vi "Read ADC.vi"(0 "Session Handle in":T1, 11 "error in (no error)":errorcluster) -> (4 "Session Handle out":T1, 6 "ADC":dbl, 8 "Error Code":string, 10 "code":i32, 15 "error out":errorcluster)   [LabVIEW 2015, in "PAS.lvclass"]
uses:
  PAS.lvclass
  Typedefs/Session Handle.ctl
panel:
  out "Success?":bool
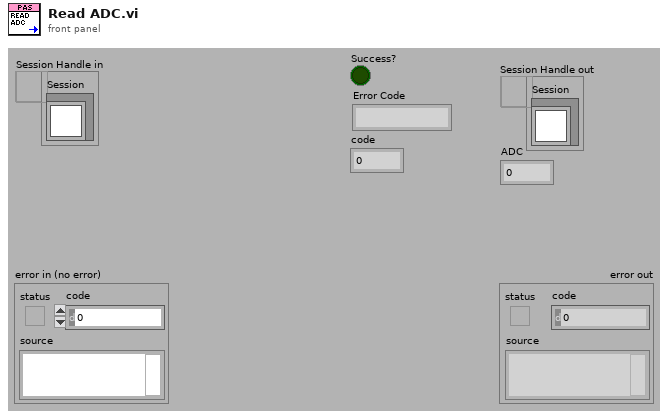
[diagram p1: front panel]
types:
  T1 = typedef "PAS.lvclass/Session Handle.ctl" = refnum<data-value>
  T2 = typedef "XNET Frame CAN.ctl" = cluster{"timestamp":timestamp, "payload":u8[], "identifier":u32, "type":T3, "extended?":bool, "echo?":bool}
  T3 = typedef "XNET Frame Type CAN.ctl" = u8
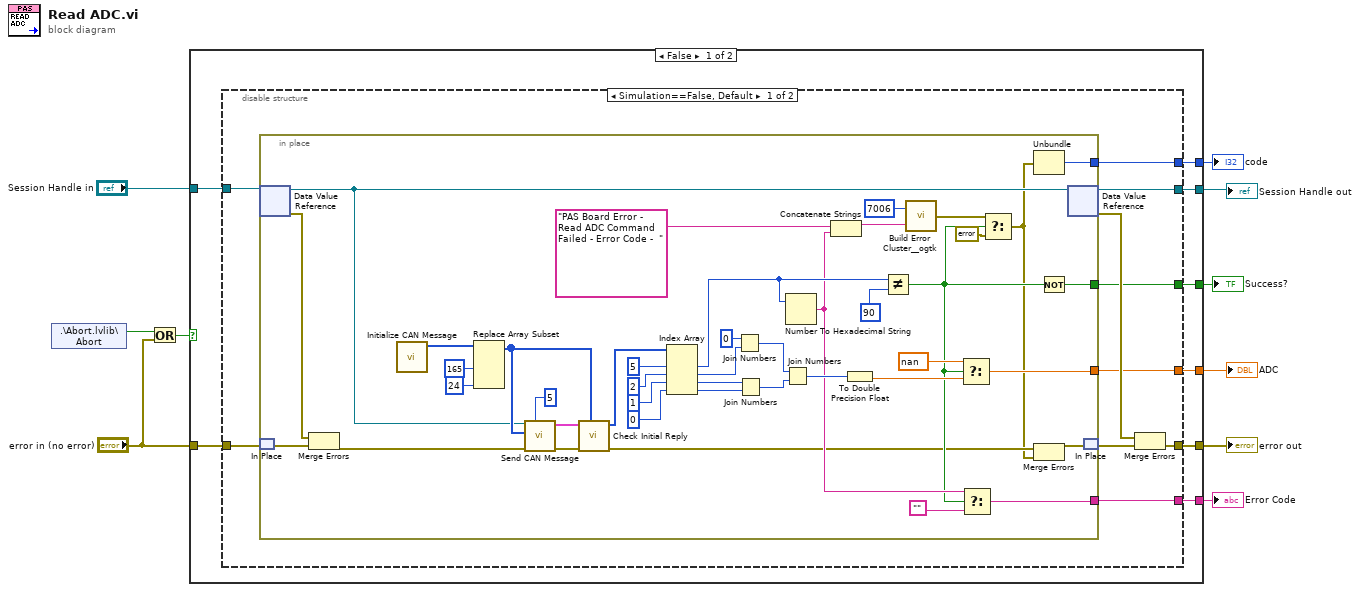
[diagram p0: block diagram]
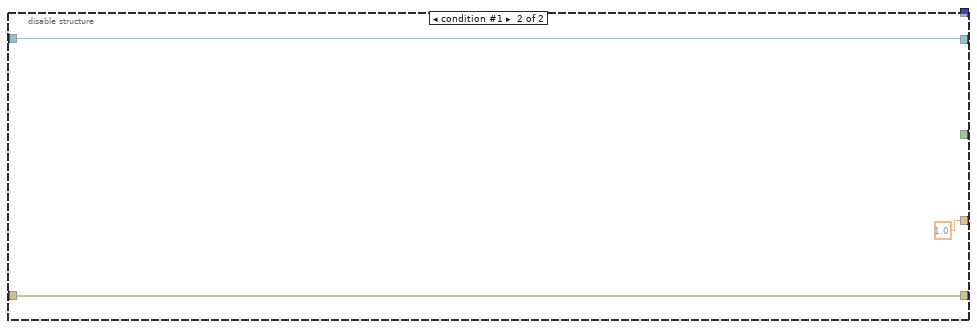
[diagram p2: hidden frame]
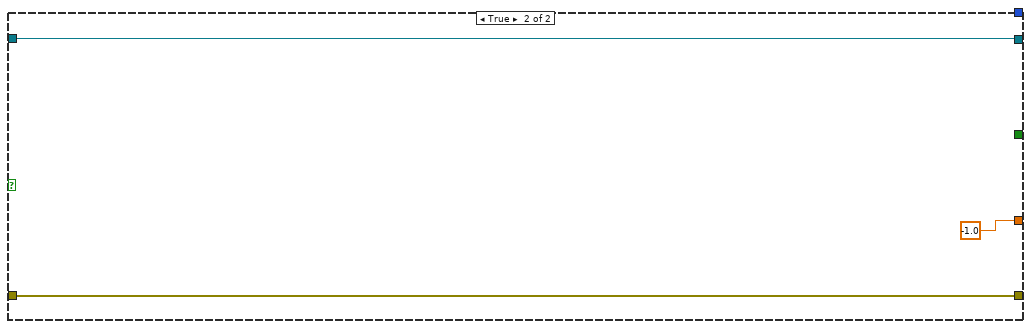
[diagram p3: hidden frame]
diagram:
  n1 = shared-variable ".\\Abort.lvlib\\Abort"() -> (w7:bool)  [unwired: 1 in, 1 out]
  n2 = Or(x=w7, y="error in (no error)") -> (x .or. y?=w5:bool)
  n3 = case shown="False" w5 {
    tunnel: [w18 w76] -> w9
    tunnel: [w17 w75] -> w8
    tunnel: "Session Handle in" -> [w16 w76]
    tunnel: "error in (no error)" -> [w15 w75]
    tunnel: [w14 -1.0] -> w4
    tunnel: [w13 _] -> w3
    tunnel: [w12 _] -> w2
    tunnel: [w11 _] -> w1
    frame False {
      n4 = disable-structure shown="Simulation==False, Default" {
        disable-tunnel: [w28 w73] -> w18
        disable-tunnel: [w25 w72] -> w17
        disable-tunnel: w16 -> [w24 w73]
        disable-tunnel: w15 -> [w23 w72]
        disable-tunnel: [w22 1.0] -> w14
        disable-tunnel: [w21 _] -> w13
        disable-tunnel: [w20 _] -> w12
        disable-tunnel: [w19 _] -> w11
        frame condition #0 (active) {
          n5 = in-place {
            in-place-border: [w48] -> w22
            in-place-border: [w54] -> w21
            in-place-border: [w33] -> w20
            in-place-border: [w29] -> w19
            n6 = in-place-dvr #1(w24) -> (w61:refnum<class "PAS.lvclass">, w66:errorcluster)
            n7 = in-place-match #2(w23) -> (w65:errorcluster)
            n8 = Merge Errors(w66, w65) -> (w60:errorcluster)
            n9 = call "Initialize CAN Message.vi"() -> ("Initial Payload"=w68:u8[])  [unwired: 11 in]
            n10 = Replace Array Subset(array=w68, new element #1=u8 165 ("new element/subarray"), new element #2=u8 24 ("new element/subarray")) -> (w64:u8[])  [unwired: 2 in]
            n11 = call "Send CAN Message.vi"("Number of Retries"=5, "error in (no error)"=w60, "payload"=w64, "Gas In"=w61) -> ("error out"=w32:errorcluster, "Reply"=w62:T2[])  [unwired: 5 in, 1 out]
            n12 = call "Check Initial Reply.vi"("Write Message"=w64, "error in (no error)"=w32, "Reply"=w62) -> ("error out"=w31:errorcluster, "Data Packet"=w67:u8[])  [unwired: 5 in, 2 out]
            n13 = Index Array(array=w67, index #1=5 ("index"), index #2=2 ("index"), index #3=1 ("index"), index #4=0 ("index")) -> (element #1=w55:u8, element #2=w43:u8, element #3=w42:u8, element #4=w41:u8)
            n14 = Join Numbers(hi=u8 0, lo=w43) -> ((hi.lo)=w40:u16)
            n15 = Join Numbers(hi=w42, lo=w41) -> ((hi.lo)=w39:u16)
            n16 = Join Numbers(hi=w40, lo=w39) -> ((hi.lo)=w38:u32)
            n17 = Number To Hexadecimal String(2:w55) -> (0:w35:string)  [unwired: 1 in]
            n18 = Concatenate Strings("PAS Board Error -  Read ADC Command Failed - Error Code -  " ("string"), w35) -> (w58:string)
            n19 = To Double Precision Float(number=w38) -> (double precision float=w37:dbl)
            n20 = Not Equal?(x=w55, y=u8 90 ("new element/subarray")) -> (x != y?=w34:bool)
            n21 = call <userlib>:"Build Error Cluster__ogtk.vi"("String to Prepend to source (\"\")"=w58, "code"=7006) -> ("error out"=w51:errorcluster)
            n22 = Select(t=nan, s=w34, f=w37) -> (s? t:f=w48:dbl)
            n23 = Select(t=w35, s=w34, f="") -> (s? t:f=w33:string)
            n24 = Select(t=w51, s=w34, f=errorcluster {"status"=FALSE, "code"=0, "source"=""}) -> (s? t:f=w30:errorcluster)
            n25 = Unbundle(w30) -> ("code"=w29:i32)  [unwired: 2 out]
            n26 = Merge Errors(w31, w30) -> (w69:errorcluster)
            n27 = Not(x=w34) -> (.not. x?=w54:bool)
            n28 = in-place-dvr #1(w61) -> (w28:T1, w26:errorcluster)
            n29 = in-place-match #2(w69) -> (w27:errorcluster)
          }
          n30 = Merge Errors(w26, w27) -> (w25:errorcluster)
        }
        frame condition #1 {
        }
      }
    }
    frame True {
    }
  }
  "Session Handle out" <- w9
  "error out" <- w8
  "ADC" <- w4
  "Success?" <- w3
  "Error Code" <- w2
  "code" <- w1
